vi "Cannon Finish.vi"   [LabVIEW 2013]
uses:
  <vilib>/Rock Robotics/WPI/Compressor/WPI_CompressorGetSetRefNum.vi
types:
  T1 = typedef "WPI_DigitalInputDevRef.ctl" = cluster{"DevStatus":errorcluster, "DIO Channel":T2, "Digital Module":T3}
  T2 = typedef "FPGA_DIOChannel.ctl" = enum8{"DIO 1", "DIO 2", "DIO 3", "DIO 4", "DIO 5", "DIO 6", "DIO 7", "DIO 8", "DIO 9", "DIO 10", "DIO 11", "DIO 12", "DIO 13", "DIO 14", "Invalid"}
  T3 = typedef "FPGA_TypedefDigitalModule.ctl" = enum16{"Digital Module 1", "Digital Module 2"}
  T4 = typedef "WPI_SolenoidDevRef.ctl" = cluster{"DevStatus":errorcluster, "Solenoid Module":T5, "Forward Solenoid Channel":T6, "Reverse Solenoid Channel":T6}
  T5 = typedef "FPGA_TypedefSolenoidModule.ctl" = enum16{"Solenoid Module 1", "Solenoid Module 2"}
  T6 = typedef "WPI_SolenoidChannel.ctl" = enum8{"Solenoid 1", "Solenoid 2", "Solenoid 3", "Solenoid 4", "Solenoid 5", "Solenoid 6", "Solenoid 7", "Solenoid 8", "Invalid"}
  T7 = typedef "WPI_CompressorDevRef.ctl" = cluster{"DevStatus":errorcluster, "DigitalInputDevRef":T1, "RelayDevRef":T8}
  T8 = typedef "WPI_RelayDevRef.ctl" = cluster{"DevStatus":errorcluster, "Relay Channel":T9, "Digital Module":T3, "Relay Direction":T10}
  T9 = typedef "FPGA_DIORelayChannel.ctl" = enum8{"Relay 1", "Relay 2", "Relay 3", "Relay 4", "Relay 5", "Relay 6", "Relay 7", "Relay 8", "Invalid"}
  T10 = typedef "WPI_RelayDirection.ctl" = enum16{"Both directions", "Forward only", "Reverse only"}
  T11 = typedef "WPI_MotorControlDeviceRef.ctl" = cluster{"DeviceStatus":errorcluster, "Type":enum16{"PWM", "CAN"}, "PWM":cluster{"Digital Module":T3, "PWM Channel":T12, "DeadBand":T13}, "CAN":cluster{"Device Number":u8, "Control Mode":T14, "Semaphore":T15, "Max Vout":dbl}, "Invert":bool, "TransformRef":T16, "InvTransformRef":T16}
  T12 = typedef "FPGA_DIOPWMChannel.ctl" = enum8{"PWM 1", "PWM 2", "PWM 3", "PWM 4", "PWM 5", "PWM 6", "PWM 7", "PWM 8", "PWM 9", "PWM 10", "Invalid"}
  T13 = typedef "WPI_PWMDeadband.ctl" = cluster{"Name":string, "maxPositivePwm":i32, "minPositivePwm":i32, "centerPwm":i32, "maxNegativePwm":i32, "minNegativePwm":i32, "angularRange":u16}
  T14 = typedef "WPI_CANJaguar_ControlMode.ctl" = enum8{"Percent VBus", "Current", "Speed", "Position", "Voltage"}
  T15 = typedef "Semaphore RefNum" = refnum<k1>
  T16 = typedef "WPI_PWMTransform_ConPane.ctl" = refnum<vi>
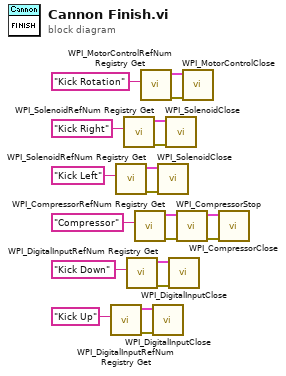
[diagram p0: block diagram]
diagram:
  n1 = call <vilib>:"WPI_DigitalInputRefNum Registry Get.vi"("refnum name"="Kick Up") -> ("error out"=w2:errorcluster, "DigitalInputDevRef"=w1:T1)  [unwired: 9 in]
  n2 = call <vilib>:"WPI_SolenoidRefNum Registry Get.vi"("refnum name"="Kick Left") -> ("error out"=w9:errorcluster, "SolenoidDevRef"=w10:T4)  [unwired: 9 in]
  n3 = call <vilib>:"WPI_SolenoidRefNum Registry Get.vi"("refnum name"="Kick Right") -> ("error out"=w12:errorcluster, "SolenoidDevRef"=w11:T4)  [unwired: 9 in]
  n4 = call <vilib>:"WPI_DigitalInputRefNum Registry Get.vi"("refnum name"="Kick Down") -> ("error out"=w4:errorcluster, "DigitalInputDevRef"=w3:T1)  [unwired: 9 in]
  n5 = call <vilib>:"WPI_CompressorRefNum Registry Get.vi"("refnum name"="Compressor") -> ("error out"=w8:errorcluster, "CompressorDevRef"=w7:T7)  [unwired: 9 in]
  n6 = call <vilib>:"WPI_MotorControlRefNum Registry Get.vi"("refnum name"="Kick Rotation") -> ("error out"=w14:errorcluster, "MotorControlDevRef"=w13:T11)  [unwired: 9 in]
  n7 = call <vilib>:"WPI_DigitalInputClose.vi"("error in (no error)"=w2, "DigitalInputDevRef"=w1) -> ()  [unwired: 9 in, 1 out]
  n8 = call <vilib>:"WPI_SolenoidClose.vi"("error in (no error)"=w9, "SolenoidDevRef"=w10) -> ()  [unwired: 9 in, 1 out]
  n9 = call <vilib>:"WPI_SolenoidClose.vi"("error in (no error)"=w12, "SolenoidDevRef"=w11) -> ()  [unwired: 9 in, 1 out]
  n10 = call <vilib>:"WPI_DigitalInputClose.vi"("error in (no error)"=w4, "DigitalInputDevRef"=w3) -> ()  [unwired: 9 in, 1 out]
  n11 = call <vilib>:"WPI_CompressorStop.vi"("error in (no error)"=w8, "CompressorDevRef"=w7) -> ("error out"=w6:errorcluster, "CompressorDevRef"=w5:T7)  [unwired: 8 in]
  n12 = call <vilib>:"WPI_MotorControlClose.vi"("error in (no error)"=w14, "MotorControlDevRef"=w13) -> ()  [unwired: 9 in, 1 out]
  n13 = call <vilib>:"WPI_CompressorClose.vi"("error in (no error)"=w6, "CompressorDevRef"=w5) -> ()  [unwired: 9 in, 1 out]
